vi "init.vi"(8 "error in":errorcluster, 10 "TBM module configuration in":refnum<class "TBM module configuration.lvclass">, 11 "Tagbus PID Module runtime in":refnum<class "PID Module runtime.lvclass">) -> (0 "error out":errorcluster, 1 "data allocations":T1, 2 "execution settings":T4, 3 "Tagbus PID Module runtime out":refnum<class "PID Module runtime.lvclass">)   [LabVIEW 2013, in "PID Module runtime.lvclass"]
doc: "Provides an interface for initializing a module at runtime. While this interface performs no operations, a child should provide an override which may open any necessary references or sessions, allocate necessary memory, and perform any final configuration validataion before providing the full configuration <b>execution data</b> to the calling process."
uses:
  PID Module runtime.lvclass
  configuration/PID Module configuration.lvclass
  <vilib>/NI/Tag Bus Module Framework/channel/TBM channel.lvclass
  <vilib>/NI/Tag Bus Module Framework/runtime/TBM module execution interface.lvclass
  <vilib>/NI/Tag Bus Module Framework/module configuration/TBM module configuration.lvclass
  <vilib>/NI/Tag Bus Module Framework/runtime/execution settings.ctl
  <vilib>/NI/Tag Bus Module Framework/channel/data tables.ctl
  <vilib>/NI/Tag Bus/dictionary/data dictionary.lvclass
  <vilib>/NI/Tag Bus/dictionary table pair.ctl
  <vilib>/NI/Tag Bus/tag bus.lvlib
  <vilib>/NI/Tag Bus/table/data table.ctl
  <vilib>/NI/Tag Bus/table/data table.lvlib
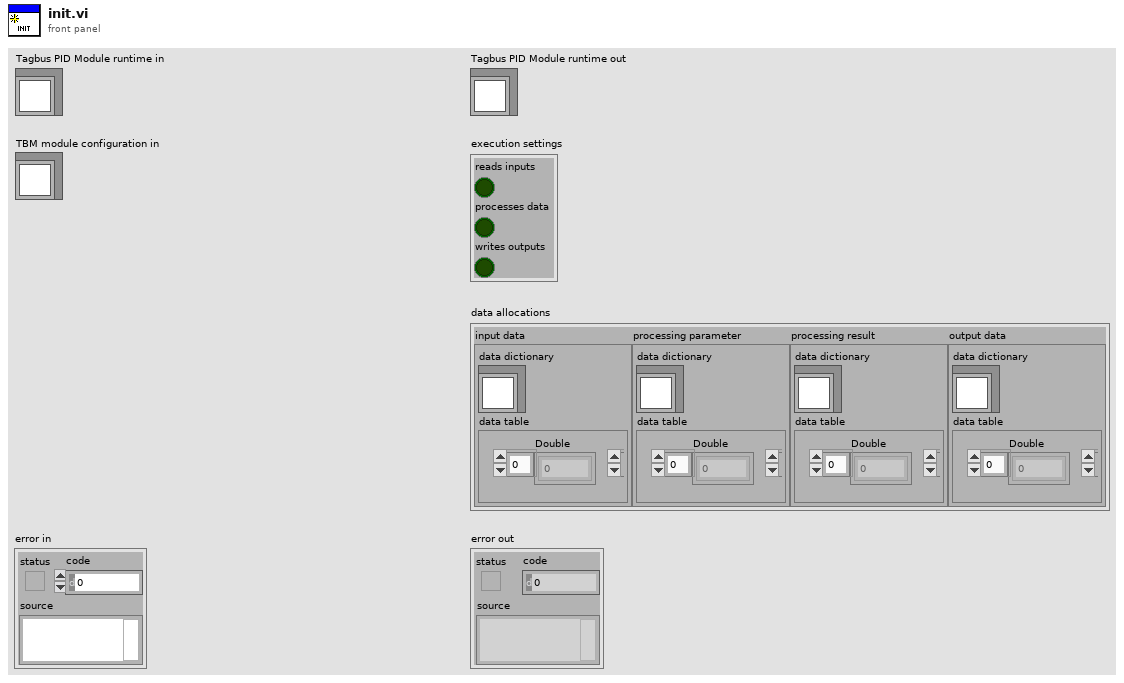
[diagram p1: front panel]
types:
  T1 = typedef "TBM channel.lvclass/data tables.ctl" = cluster{"input data":T2, "processing parameter":T2, "processing result":T2, "output data":T2}
  T2 = typedef "tag bus.lvlib/dictionary table pair.ctl" = cluster{"data dictionary":refnum<class "data dictionary.lvclass">, "data table":T3}
  T3 = typedef "tag bus.lvlib/data table.lvlib/data table.ctl" = cluster{"Double":dbl[], "Single":sgl[], "I64":i64[], "I32":i32[], "I16":i16[], "I8":i8[], "U64":u64[], "U32":u32[], "U16":u16[], "U8":u8[], "Boolean":bool[], "String":string[], "Array of Double":cluster{"DBL Array":dbl[]}[], "Array of Single":cluster{"SGL Array":sgl[]}[], "Array of I64":cluster{"I64 Array":i64[]}[], "Array of I32":cluster{"I32 Array":i32[]}[], "Array of I16":cluster{"I16 Array":i16[]}[], "Array of I8":cluster{"I8 Array":i8[]}[], "Array of U64":cluster{"U64 Array":u64[]}[], "Array of U32":cluster{"U32 Array":u32[]}[], "Array of U16":cluster{"U16 Array":u16[]}[], "Array of U8":cluster{"U8 Array":u8[]}[], "Array of Boolean":cluster{"Boolean Array":bool[]}[], "Array of String":cluster{"String Array":string[]}[]}
  T4 = typedef "TBM module execution interface.lvclass/execution settings.ctl" = cluster{"reads inputs":bool, "processes data":bool, "writes outputs":bool}
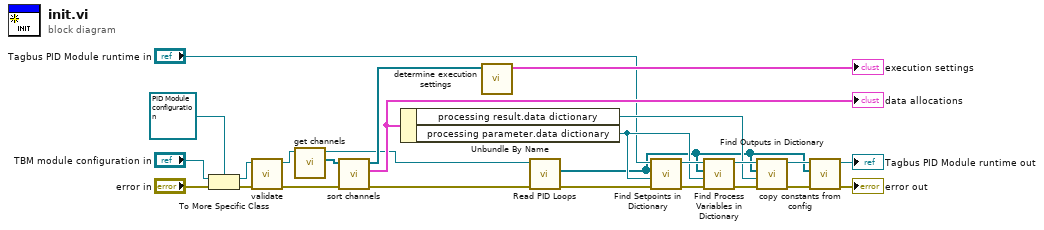
[diagram p0: block diagram]
diagram:
  n1 = To More Specific Class(target class=refnum<class "PID Module configuration.lvclass"> refnum ("Synchronous module configuration"), reference="TBM module configuration in", error in="error in") -> (specific class reference=w25:refnum<class "PID Module configuration.lvclass">, error out=w26:errorcluster)
  n2 = call-dynamic "validate.vi"("error in"=w26, "Tagbus PID Module configuration in"=w25) -> ("error out"=w20:errorcluster, "Tagbus PID Module configuration out"=w19:refnum<class "PID Module configuration.lvclass">)  [unwired: 8 in]
  n3 = call-dynamic "get channels.vi"("module configuration in"=w19) -> ("channels"=w18:refnum<class "TBM channel.lvclass">[], "module configuration out"=w15:refnum<class "PID Module configuration.lvclass">)  [unwired: 9 in]
  n4 = call <vilib>:"sort channels.vi"("error in"=w20, "channels in"=w18) -> ("error out"=w14:errorcluster, "data allocations"=w17:T1, "channels out"=w16:refnum<class "TBM channel.lvclass">[])  [unwired: 7 in]
  "data allocations" <- w17
  n5 = Unbundle By Name(w17) -> ("processing result.data dictionary"=w8:refnum<class "data dictionary.lvclass">, "processing parameter.data dictionary"=w7:refnum<class "data dictionary.lvclass">)
  n6 = call <vilib>:"determine execution settings.vi"("channels"=w16) -> ("execution settings"=→"execution settings":T4)  [unwired: 10 in]
  n7 = call-dynamic "Read PID Loops.vi"("error in (no error)"=w14, "Tagbus PID Module configuration in"=w15) -> ("error out"=w13:errorcluster, "PID Loops"=w1:refnum<class "PID Loop.lvclass">[])  [unwired: 7 in, 1 out]
  n8 = call-dynamic "Find Setpoints in Dictionary.vi"("error in (no error)"=w13, "processing data dictionary"=w7, "PID Loops in"=w1, "Tagbus PID Module runtime"="Tagbus PID Module runtime in") -> ("error out"=w11:errorcluster, "Tagbus PID Module output"=w12:refnum<class "PID Module runtime.lvclass">)  [unwired: 6 in]
  n9 = call-dynamic "Find Process Variables in Dictionary.vi"("error in (no error)"=w11, "processing data dictionary"=w7, "PID Loops"=w1, "Tagbus PID Module runtime in"=w12) -> ("error out"=w10:errorcluster, "Tagbus PID Module runtime out"=w9:refnum<class "PID Module runtime.lvclass">)  [unwired: 6 in]
  n10 = call-dynamic "Find Outputs in Dictionary.vi"("error in (no error)"=w10, "processing data dictionary"=w8, "PID Loops"=w1, "Tagbus PID Module runtime in"=w9) -> ("error out"=w4:errorcluster, "Tagbus PID Module runtime out"=w6:refnum<class "PID Module runtime.lvclass">)  [unwired: 6 in]
  n11 = call-dynamic "copy constants from config.vi"("error in (no error)"=w4, "PID Loops"=w1, "Tagbus PID Module runtime in"=w6) -> ("error out"=→"error out":errorcluster, "Tagbus PID Module runtime out"=→"Tagbus PID Module runtime out":refnum<class "PID Module runtime.lvclass">)  [unwired: 7 in]
